vi "数据处理直接插入整合 (子VI).vi"   [LabVIEW 2016, in "数据传输系统-05.lvlib"]
types:
  T1 = cluster{"PH":string[][], "CODCr":string[][], "氨氮":string[][], "CODMn":string[][], "总氮":string[][], "总磷":string[][], "电导率":string[][], "水温":string[][], "DO":string[][], "浊度":string[][], "叶绿素":string[][], "藻密度":string[][], "铜":string[][], "盐度":string[][], "水位":string[][], "流速":string[][], "瞬时流量":string[][], "累积流量":string[][], "亚硝酸盐":string[][], "硫化物":string[][], "ORP":string[][], "铅":string[][], "镉":string[][], "锌":string[][], "镍":string[][], "锰":string[][], "汞":string[][], "气温":string[][], "气压":string[][], "风速":string[][], "风向":string[][], "盐度 2":string[][], "磷酸盐":string[][], "硝氮":string[][], "氟化物":string[][]}
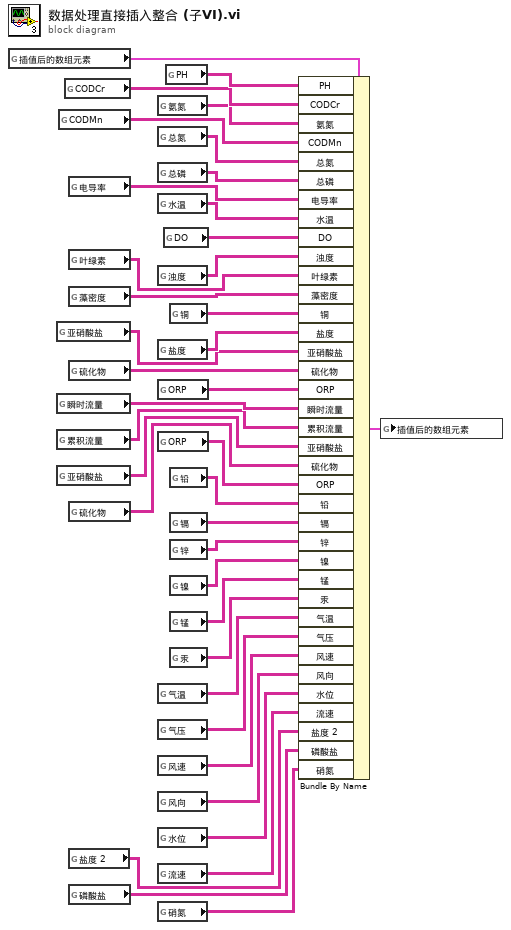
[diagram p0: block diagram]
diagram:
  n1 = global read "插值后的新数组.vi" "插值后的数组元素"() -> (w25:T1)
  n2 = global read "全局 所有参数.vi" "亚硝酸盐"() -> (w22:string[][])
  n3 = global read "全局 所有参数.vi" "瞬时流量"() -> (w20:string[][])
  n4 = global read "全局 所有参数.vi" "累积流量"() -> (w19:string[][])
  n5 = global read "全局 所有参数.vi" "亚硝酸盐"() -> (w18:string[][])
  n6 = global read "全局 所有参数.vi" "CODMn"() -> (w36:string[][])
  n7 = global read "全局 所有参数.vi" "CODCr"() -> (w38:string[][])
  n8 = global read "全局 所有参数.vi" "电导率"() -> (w33:string[][])
  n9 = global read "全局 所有参数.vi" "叶绿素"() -> (w29:string[][])
  n10 = global read "全局 所有参数.vi" "藻密度"() -> (w28:string[][])
  n11 = global read "全局 所有参数.vi" "硫化物"() -> (w23:string[][])
  n12 = global read "全局 所有参数.vi" "硫化物"() -> (w17:string[][])
  n13 = global read "全局 所有参数.vi" "盐度 2"() -> (w3:string[][])
  n14 = global read "全局 所有参数.vi" "磷酸盐"() -> (w2:string[][])
  n15 = global read "全局 所有参数.vi" "氨氮"() -> (w37:string[][])
  n16 = global read "全局 所有参数.vi" "总氮"() -> (w35:string[][])
  n17 = global read "全局 所有参数.vi" "总磷"() -> (w34:string[][])
  n18 = global read "全局 所有参数.vi" "水温"() -> (w32:string[][])
  n19 = global read "全局 所有参数.vi" "浊度"() -> (w30:string[][])
  n20 = global read "全局 所有参数.vi" "盐度"() -> (w26:string[][])
  n21 = global read "全局 所有参数.vi" "ORP"() -> (w24:string[][])
  n22 = global read "全局 所有参数.vi" "ORP"() -> (w16:string[][])
  n23 = global read "全局 所有参数.vi" "气温"() -> (w9:string[][])
  n24 = global read "全局 所有参数.vi" "气压"() -> (w8:string[][])
  n25 = global read "全局 所有参数.vi" "风速"() -> (w7:string[][])
  n26 = global read "全局 所有参数.vi" "风向"() -> (w6:string[][])
  n27 = global read "全局 所有参数.vi" "水位"() -> (w5:string[][])
  n28 = global read "全局 所有参数.vi" "流速"() -> (w4:string[][])
  n29 = global read "全局 所有参数.vi" "硝氮"() -> (w1:string[][])
  n30 = global read "全局 所有参数.vi" "DO"() -> (w31:string[][])
  n31 = global read "全局 所有参数.vi" "PH"() -> (w39:string[][])
  n32 = global read "全局 所有参数.vi" "铜"() -> (w27:string[][])
  n33 = global read "全局 所有参数.vi" "铅"() -> (w15:string[][])
  n34 = global read "全局 所有参数.vi" "镉"() -> (w14:string[][])
  n35 = global read "全局 所有参数.vi" "锌"() -> (w13:string[][])
  n36 = global read "全局 所有参数.vi" "镍"() -> (w12:string[][])
  n37 = global read "全局 所有参数.vi" "锰"() -> (w11:string[][])
  n38 = global read "全局 所有参数.vi" "汞"() -> (w10:string[][])
  n39 = Bundle By Name(cluster=w25, "PH"=w39, "CODCr"=w38, "氨氮"=w37, "CODMn"=w36, "总氮"=w35, "总磷"=w34, "电导率"=w33, "水温"=w32, "DO"=w31, "浊度"=w30, "叶绿素"=w29, "藻密度"=w28, "铜"=w27, "盐度"=w26, "亚硝酸盐"=w22, "硫化物"=w23, "ORP"=w24, "瞬时流量"=w20, "累积流量"=w19, "亚硝酸盐"=w18, "硫化物"=w17, "ORP"=w16, "铅"=w15, "镉"=w14, "锌"=w13, "镍"=w12, "锰"=w11, "汞"=w10, "气温"=w9, "气压"=w8, "风速"=w7, "风向"=w6, "水位"=w5, "流速"=w4, "盐度 2"=w3, "磷酸盐"=w2, "硝氮"=w1) -> (w21:T1)
  n40 = global write "插值后的新数组.vi" "插值后的数组元素"(w21) -> ()
